vi "GUI_DG645_2.0.0.vi"() -> ()   [LabVIEW 2013]
uses:
  DelayControl_For Multiple Channels.ctl
  Device Drivers/DG645/subVIs/channels_TypDef.ctl
  DelayControl2.ctl
  Device Drivers/DG645/subVIs/polarity_TypDEf.ctl
  Shared/GUI_Template/GUI_master/tcp_new_data_event.ctl
  Shared/GUI_Template/GUI_master/tcp new data cluster.ctl
panel:
  out "tcp data event":T1
  in  "Refresh Button":bool
  in  "GUIdevice 1":string="P2-AndorCam"
  out "UDP error message":string caption="Device Errors"
  in  "Plot":bool
  in  "Tab Control":enum32{"All Channels", "Internal", "Advanced"}(tab)
  out "Plot Array":cluster{"Waveform Graph":dbl[]}[](array[cluster])
  in  "Amplitude.Ch GH::1":dbl=4.0 caption="Amplitude (V)" min=0.5 max=5.0
  in  "Amplitude.Ch T0::1":dbl=4.0 caption="Amplitude (V)" min=0.5 max=5.0
  in  "Polarity.Ch GH::1":T2=enum."Positive" caption="Polarity"
  in  "Polarity.Ch T0::1":T2=enum."Positive" caption="Polarity"
  in  "Delay.Ch T1":T3={"Channel"="T1", "Linked"=enum."T0", "Delay"=0.03} {"Delay" format="%+.12f"}
  in  "Delay.Ch T0":T3={"Channel"="T0", "Linked"=enum."T0", "Delay"=0.0} {"Delay" format="%+.12f"}
  in  "Delay.Ch H":T3={"Channel"="H", "Linked"=enum."G", "Delay"=0.03} {"Delay" format="%+.12f"}
  in  "Delay.Ch G":T3={"Channel"="G", "Linked"=enum."T0", "Delay"=0.0} {"Delay" format="%+.12f"}
  in  "Polarity.Ch EF::1":T2=enum."Positive" caption="Polarity"
  in  "Amplitude.Ch EF::1":dbl=4.0 caption="Amplitude (V)" min=0.5 max=5.0
  in  "Delay.Ch F":T3={"Channel"="F", "Linked"=enum."E", "Delay"=0.03} {"Delay" format="%+.12f"}
  in  "Delay.Ch E":T3={"Channel"="E", "Linked"=enum."T0", "Delay"=0.0} {"Delay" format="%+.12f"}
  in  "Polarity.Ch CD::1":T2=enum."Positive" caption="Polarity"
  in  "Amplitude.Ch CD::1":dbl=4.0 caption="Amplitude (V)" min=0.5 max=5.0
  in  "Delay.Ch D":T3={"Channel"="D", "Linked"=enum."C", "Delay"=0.03} {"Delay" format="%+.12f"}
  in  "Delay.Ch C":T3={"Channel"="C", "Linked"=enum."T0", "Delay"=0.0} {"Delay" format="%+.12f"}
  in  "Delay.Ch B":T3={"Channel"="B", "Linked"=enum."A", "Delay"=0.03} {"Delay" format="%+.12f"}
  in  "Delay.Ch A":T3={"Channel"="A", "Linked"=enum."T0", "Delay"=0.0} {"Delay" format="%+.12f"}
  in  "Amplitude.Ch AB:::1":dbl=3.0 caption="Amplitude (V)"
  in  "Polarity.Ch AB::1":T2=enum."Positive" caption="Polarity"
  in  "local saving path::1":path caption="Local Saving Path"
  in  "load file::1":bool caption="Load file"
  in  "save::1":bool caption="save"
  in  "trigger::1":bool caption="Trigger"
  in  "load local::1":T6(ring) caption="load local"
  in  "save local::1":T6(ring) caption="save local"
  in  "trigger.rate::1":dbl=10.0 caption="Rate (Hz)" min=0.001 max=1000.0
  in  "trigger.source::1":T7(ring)=enum."External rising edges" caption="Source"
  in  "Inhibit::1":T8(ring)=enum."Triggers" caption="Inhibit"
  in  "stop":bool
  # "AB"
  # "CD"
  # "EF"
  # "GH"
  # "T0"
  # "="
  # "="
  # "="
  # "="
  # "="
  # "="
  # "="
  # "="
  # "="
  # "="
  # "TRIGGER"
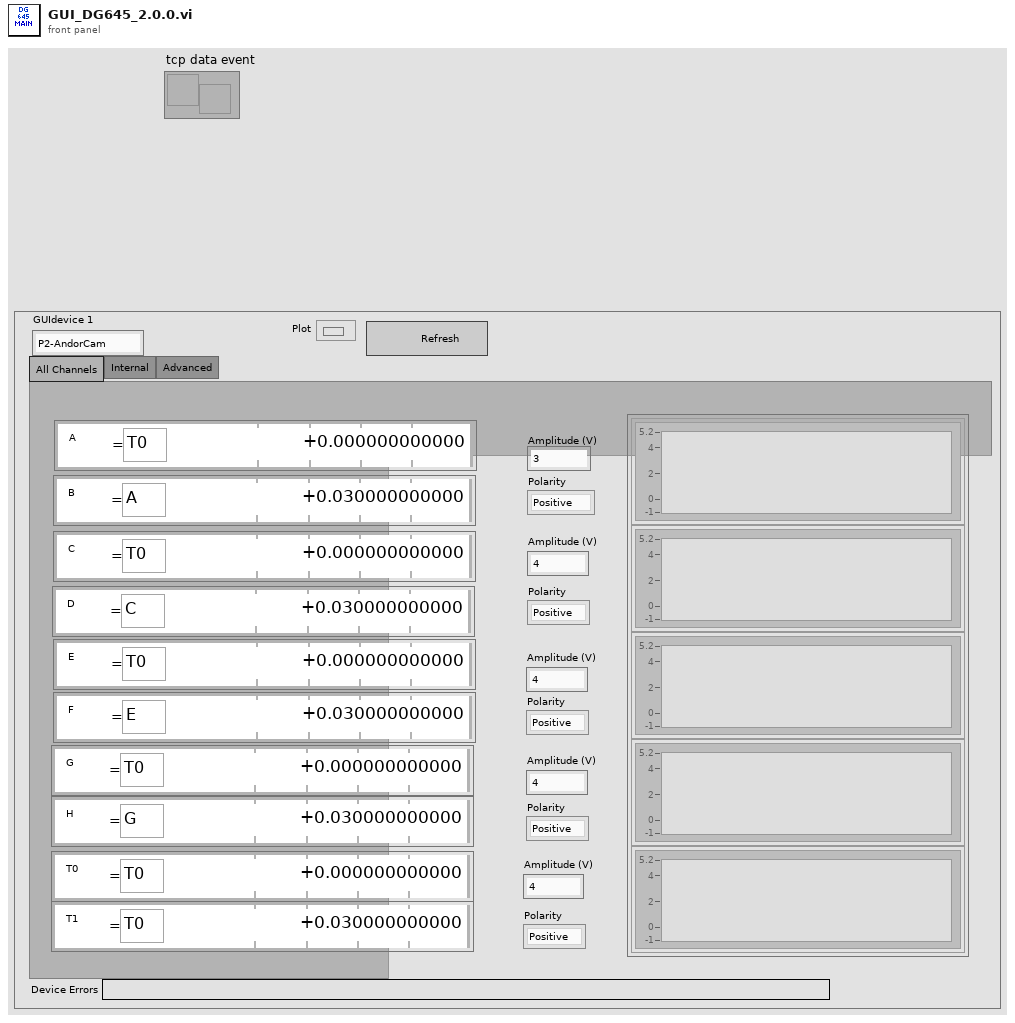
[diagram p1: front panel]
types:
  T1 = typedef "tcp_new_data_event.ctl" = refnum<user-event>
  T2 = typedef "polarity_TypDEf.ctl" = enum16{"Negative", "Positive"}
  T3 = typedef "DelayControl_For Multiple Channels.ctl" = cluster{"Channel":string, "Linked":T4, "Delay":T5}
  T4 = typedef "channels_TypDef.ctl" = enum16{"T0", "T1", "A", "B", "C", "D", "E", "F", "G", "H"}
  T5 = typedef "DelayControl2.ctl" = dbl
  T6 = enum16{"off", "1", "2", "3", "4", "5", "6", "7", "8", "9"}
  T7 = enum16{"Internal", "External rising edges", "External falling edges", "Single shot external rising edges", "Single shot external falling edges", "Single shot", "Line"}
  T8 = enum16{"off", "Triggers", "AB", "AB and CD", "AB, CD and EF", "AB, CD, EF and GH"}
  T9 = enum32{"invalid app kind", "Development System", "Run Time System", "Student Edition", "Embedded LabVIEW", "Evaluation", "Custom"}
  T10 = typedef "tcp new data cluster.ctl" = cluster{"EventEnum":enum16{"new data", "connection status update"}, "Device name":string}
  T11 = enum32{"Invalid", "Standard", "Closed", "Hidden", "Minimized", "Maximized"}
  T12 = cluster{"Core":cluster{"Current VI Reference":refnum<vi>, "Close Panel on Exit?":bool}, "Your Boolean data":bool, "Your string data":string, "SuperGUI":cluster{"STOP queue":refnum<queue>, "SuperGUI ref":refnum<vi>}}
  T13 = cluster{"STOP queue":refnum<queue>, "SuperGUI ref":refnum<vi>}
  T14 = cluster{"Current VI Reference":refnum<vi>, "Close Panel on Exit?":bool}
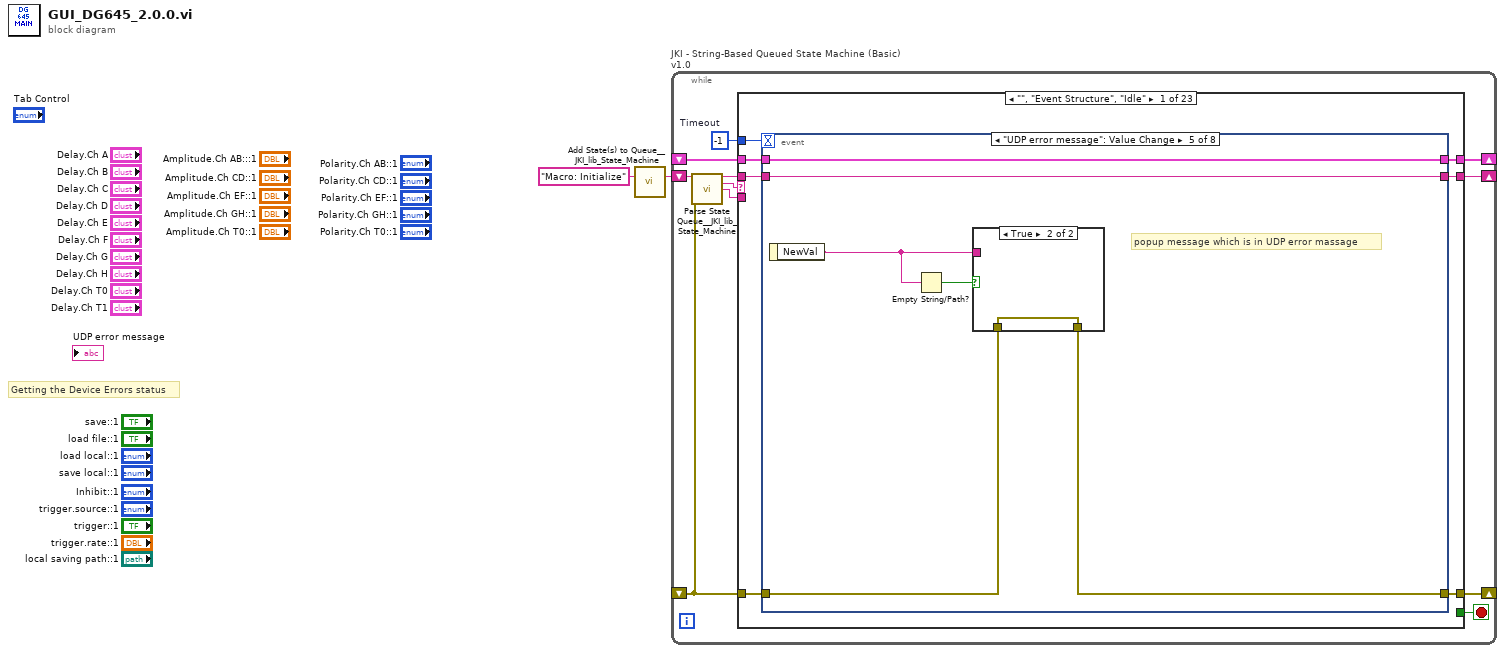
[diagram p0: block diagram]
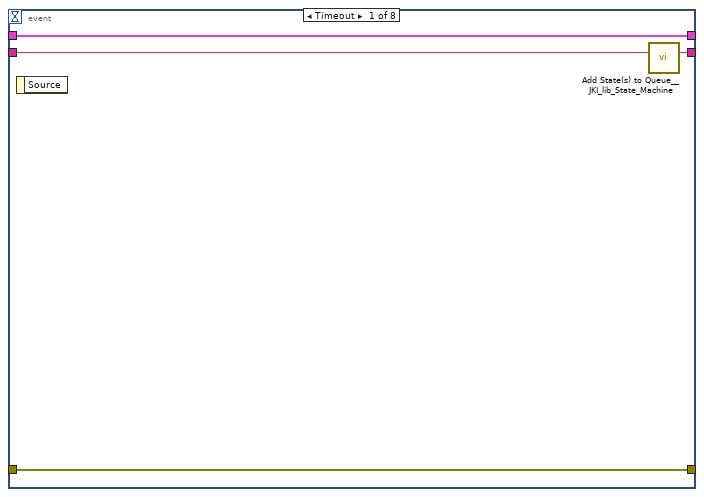
[diagram p2: hidden frame]
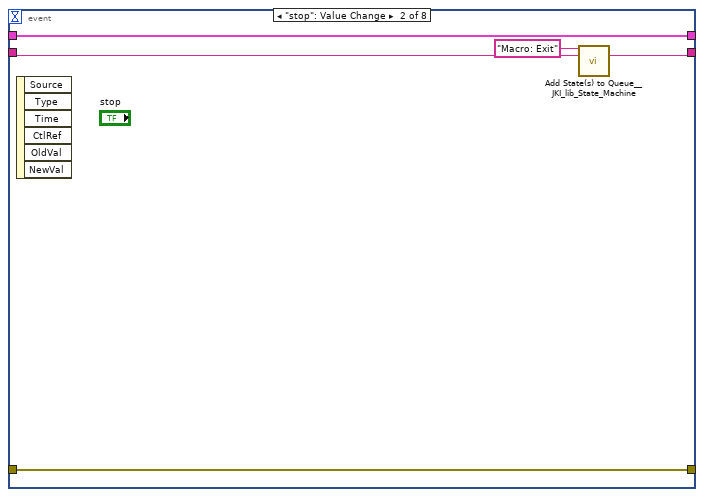
[diagram p3: hidden frame]
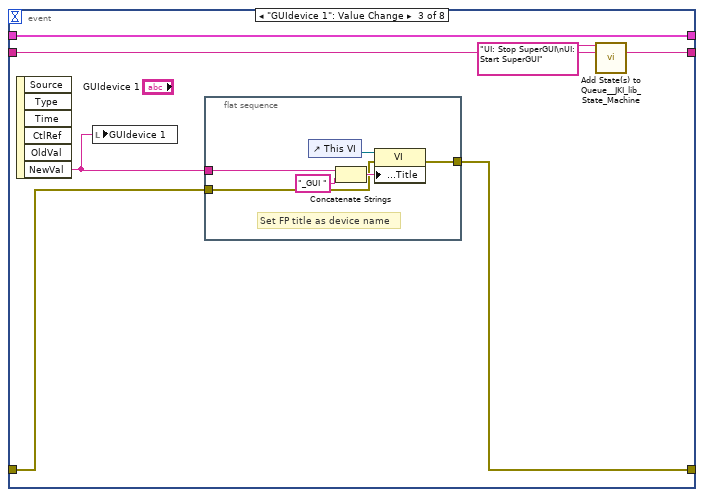
[diagram p4: hidden frame]
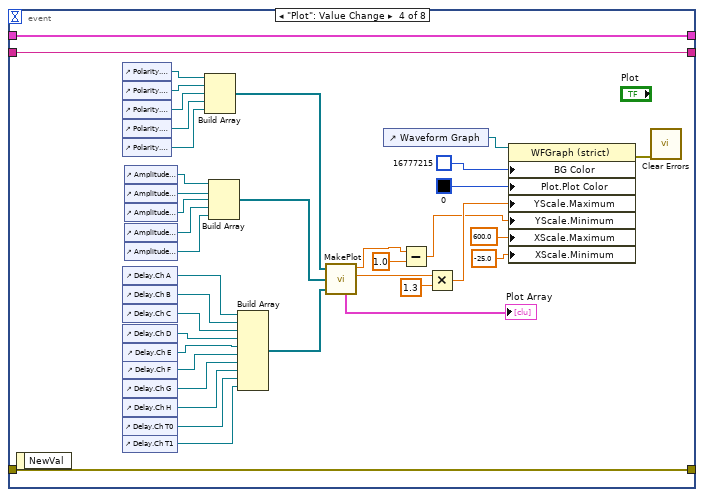
[diagram p5: hidden frame]
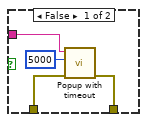
[diagram p6: hidden frame]
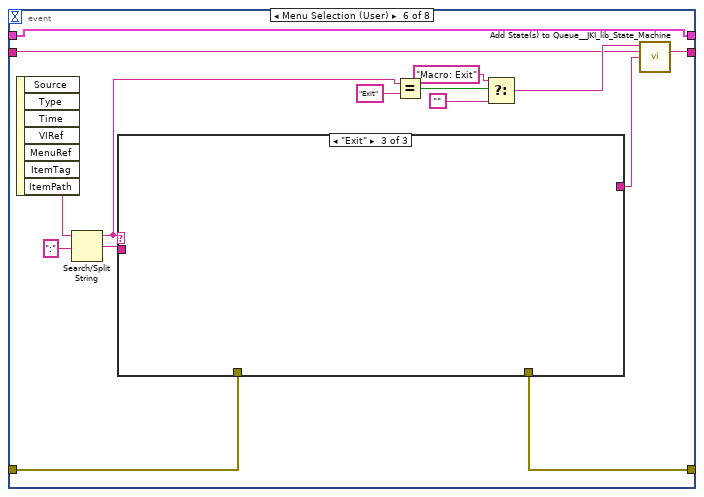
[diagram p7: hidden frame]
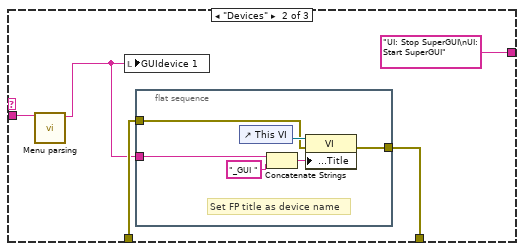
[diagram p9: hidden frame]
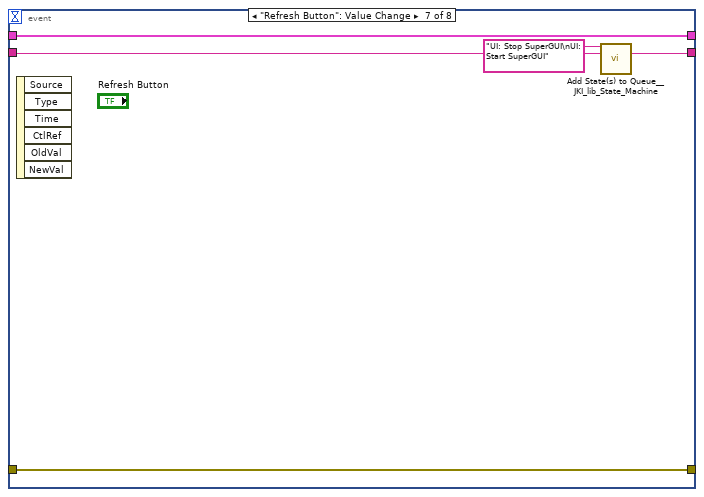
[diagram p10: hidden frame]
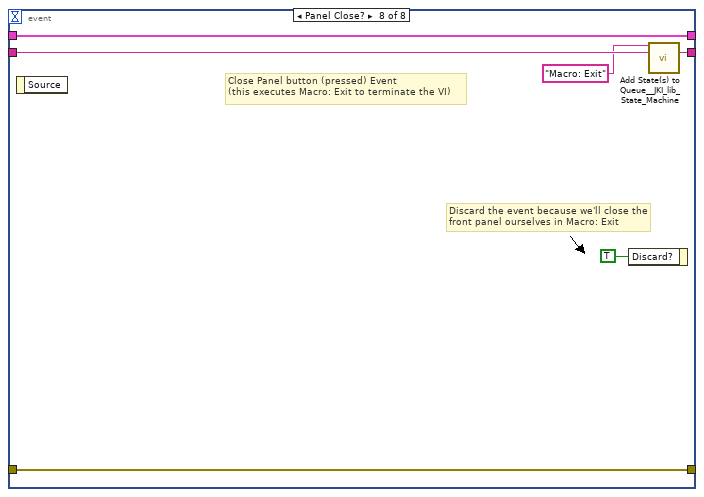
[diagram p11: hidden frame]
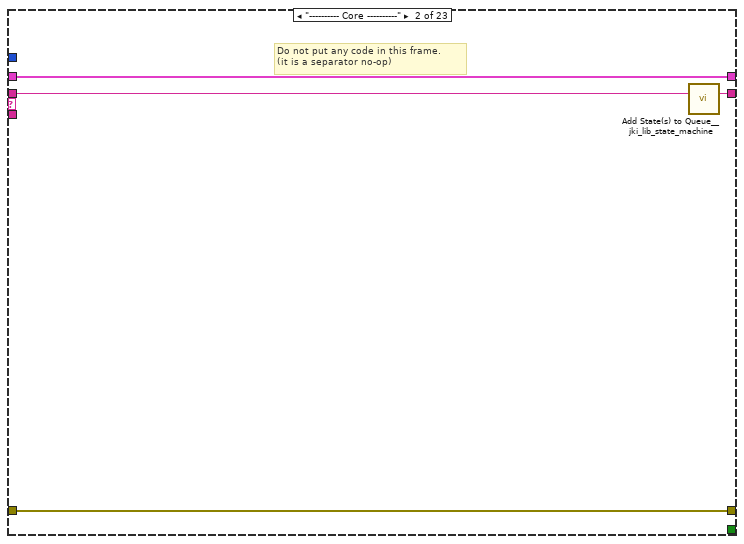
[diagram p12: hidden frame]
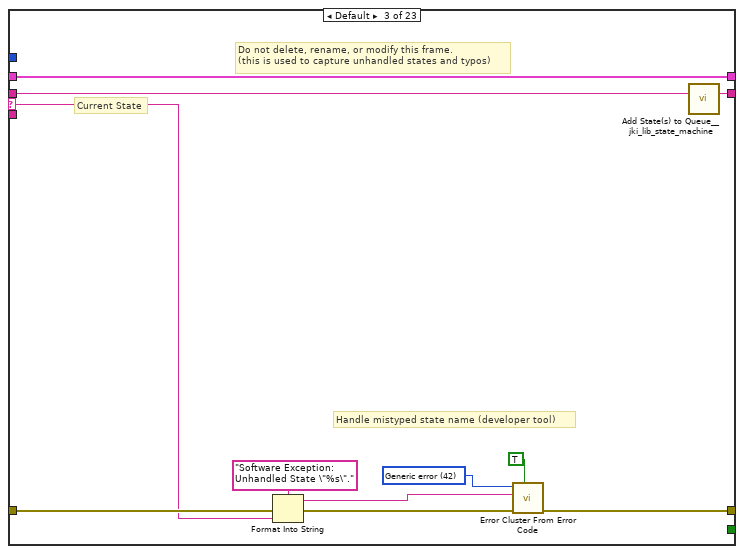
[diagram p13: hidden frame]
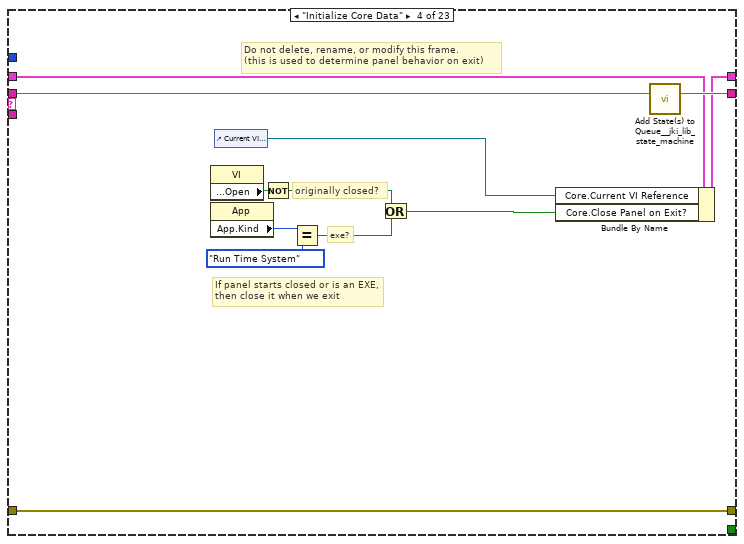
[diagram p14: hidden frame]
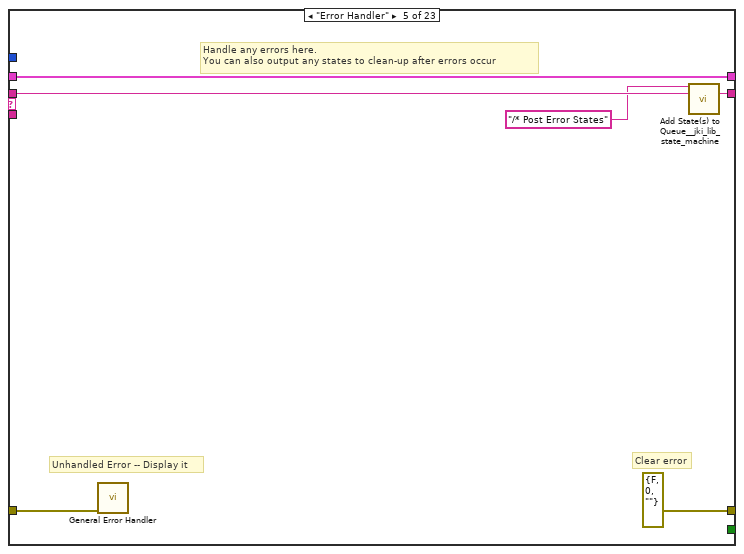
[diagram p15: hidden frame]
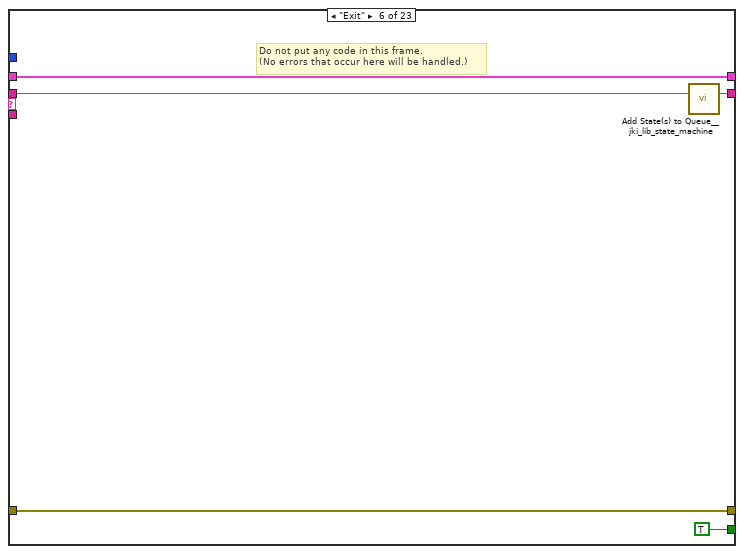
[diagram p16: hidden frame]
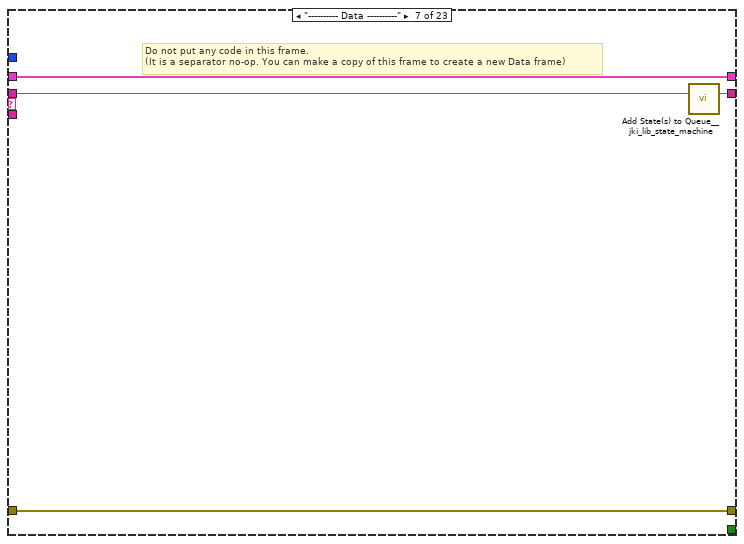
[diagram p17: hidden frame]
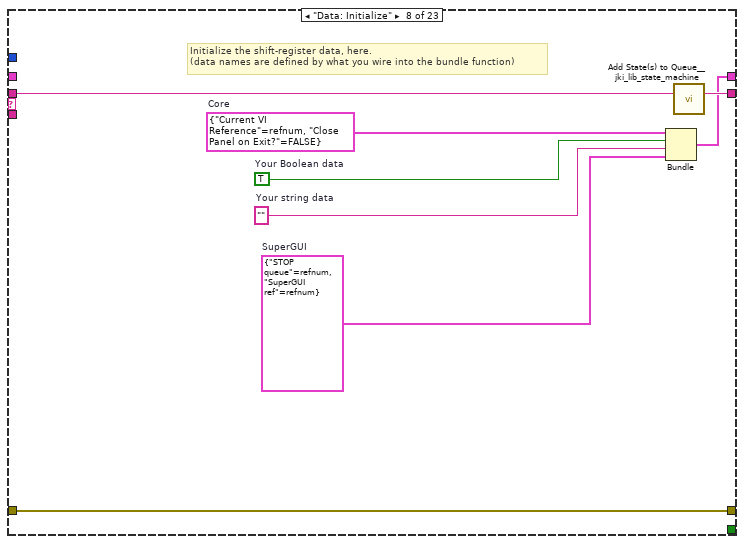
[diagram p18: hidden frame]
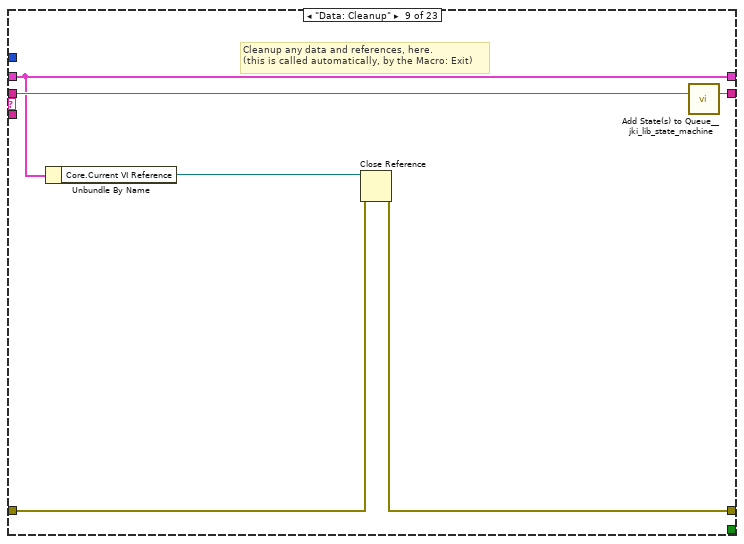
[diagram p19: hidden frame]
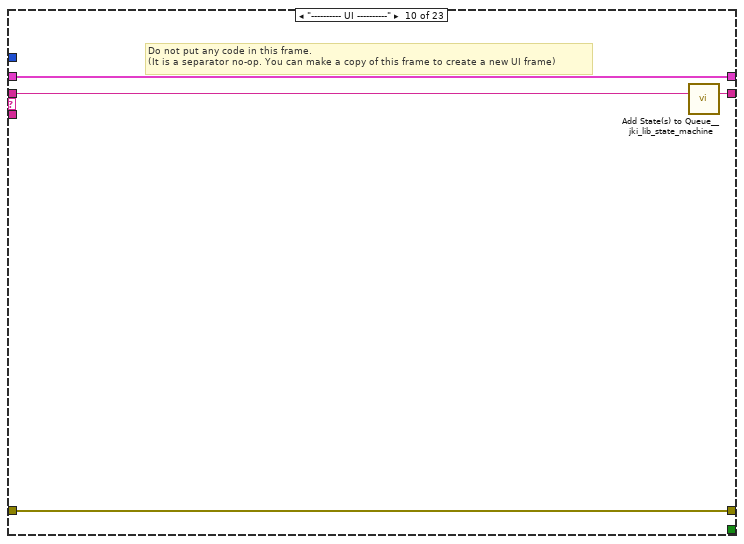
[diagram p20: hidden frame]
diagram:
  # "Getting the Device Errors status"
  n1 = call <vilib>:"Add State(s) to Queue__JKI_lib_State_Machine.vi"("State(s) in (\"\")"="Macro: Initialize") -> ("States Out"=w2:string)  [unwired: 14 in]
  n2 = while "JKI - String-Based Queued State Machine (Basic) v1.0" {
    shift-right: [w6] -> _
    shift-left: _ -> [w5]
    shift-right: [w9] -> _
    shift-left: _ -> [w3]
    shift-right: [w8] -> _
    shift-left: w2 -> [w10]
    stop <- w7 stop-if-true
    w4 = -1  # Timeout
    n3 = call <vilib>:"Parse State Queue__JKI_lib_State_Machine.vi"("State Queue"=w10, "Error In (no error)"=w3) -> ("Remaining States"=w12:string, "Current State"=w13:string, "Arguments"=w11:string)  [unwired: 11 in]
    n4 = case shown="\"\", \"Event Structure\", \"Idle\"" w13 {
      selector: w13 -> [_ _ w136 _ _ _ _ _ _ _ _ _ _ _ _ _ _ _ _ _ _ _ _]
      tunnel: w12 -> [w20 w135 w140 w158 w164 w169 w173 w181 w187 w191 w196 w204 w236 w270 w278 w284 w295 w321 w326 w336 w340 w344 w348]
      tunnel: w11 -> [_ _ _ _ _ _ _ _ _ _ _ _ _ _ _ w279 w289 _ _ _ _ _ _]
      tunnel: w5 -> [w18 w132 w138 w149 w161 w167 w170 _ w182 w188 w194 w202 w234 w261 w273 w282 w291 w318 w323 w333 w337 w341 w345]
      tunnel: [w17 w133 w142 w155 errorcluster {"status"=FALSE, "code"=0, "source"=""} ("error out") w166 w171 w178 w183 w189 w192 w200 w231 w254 w271 w280 w292 w319 w324 w334 w338 w342 w346] -> w9
      tunnel: w3 -> [w16 w133 w141 w155 w160 w166 w171 w178 w184 w189 w193 w201 w232 w255 w272 w281 w293 w319 w324 w334 w338 w342 w346]
      tunnel: [w19 w134 w139 w157 w163 w168 w172 w180 w186 w190 w195 w203 w235 w269 w277 w283 w294 w320 w325 w335 w339 w343 w347] -> w8
      tunnel: [_ _ _ _ _ TRUE _ _ _ _ _ _ _ _ _ _ _ _ _ _ _ _ _] -> w7
      tunnel: [w15 w132 w138 w156 w161 w167 w170 w179 w182 w188 w194 w202 w234 w260 w273 w282 w291 w318 w323 w333 w337 w341 w345] -> w6
      tunnel: w4 -> [w14 _ _ _ _ _ _ _ _ _ _ _ _ _ _ _ _ _ _ _ _ _ _]
      frame "", "Event Structure", "Idle" {
        n5 = event shown="[4] \"UDP error message\": Value Change" {
          selector: _ -> [_ _ _ _ _ _ _ _]
          dyn-events: _ -> [_ _ _ _ _ _ _ _]
          timeout: w14 -> [_ _ _ _ _ _ _ _]
          tunnel: w20 -> [w24 w27 w33 w80 w86 w101 w123 w131]
          tunnel: [w23 w26 w32 w80 w86 w100 w122 w130] -> w19
          tunnel: w18 -> [w21 w29 w36 w81 w87 w107 w125 w128]
          tunnel: [w22 w28 w34 w79 w82 w94 w124 w129] -> w17
          tunnel: w16 -> [w22 w28 w35 w79 w83 w95 w124 w129]
          tunnel: [w21 w29 w36 w81 w87 w107 w125 w128] -> w15
          event Timeout {
            n6 = event-data() -> ()  [unwired: 1 in, 1 out]
            n7 = call <vilib>:"Add State(s) to Queue__JKI_lib_State_Machine.vi"("State(s) in (\"\")"=w24) -> ("States Out"=w23:string)  [unwired: 14 in]
          }
          event "stop": Value Change {
            n8 = event-data() -> ()  [unwired: 1 in, 6 out]
            n9 = call <vilib>:"Add State(s) to Queue__JKI_lib_State_Machine.vi"("State(s) in Front (\"\")"="Macro: Exit", "State(s) in (\"\")"=w27) -> ("States Out"=w26:string)  [unwired: 13 in]
          }
          event "GUIdevice 1": Value Change {
            n10 = event-data() -> ("NewVal"=w30:string)  [unwired: 1 in, 5 out]
            n11 = local write "GUIdevice 1"(w30) -> ()
            n12 = flat-sequence {
              tunnel: [w39] -> w34
              tunnel: w35 -> [w38]
              tunnel: w30 -> [w37]
              frame #0 {
                # "Set FP title as device name"
                n13 = control-ref of="This VI"() -> (w42:refnum<vi>)
                n14 = Concatenate Strings(w37, "_GUI ") -> (w41:string)
                n15 = property class="VI"(reference=w42, error in=w38, "Front Panel.Title"=w41) -> (error out=w39:errorcluster)  [unwired: 1 out]
              }
            }
            n16 = call <vilib>:"Add State(s) to Queue__JKI_lib_State_Machine.vi"("State(s) in Front (\"\")"="UI: Stop SuperGUI\nUI: Start SuperGUI", "State(s) in (\"\")"=w33) -> ("States Out"=w32:string)  [unwired: 13 in]
          }
          event "Plot": Value Change {
            n17 = event-data() -> ()  [unwired: 1 in, 1 out]
            n18 = control-ref of="Polarity.Ch AB"() -> (w65:refnum<vi>)
            n19 = control-ref of="Polarity.Ch CD"() -> (w64:refnum<vi>)
            n20 = control-ref of="Polarity.Ch EF"() -> (w63:refnum<vi>)
            n21 = control-ref of="Polarity.Ch GH"() -> (w62:refnum<vi>)
            n22 = control-ref of="Polarity.Ch T0"() -> (w61:refnum<vi>)
            n23 = control-ref of="Delay.Ch A"() -> (w53:refnum<vi>)
            n24 = control-ref of="Delay.Ch B"() -> (w52:refnum<vi>)
            n25 = control-ref of="Delay.Ch C"() -> (w51:refnum<vi>)
            n26 = control-ref of="Delay.Ch D"() -> (w50:refnum<vi>)
            n27 = control-ref of="Delay.Ch E"() -> (w49:refnum<vi>)
            n28 = control-ref of="Delay.Ch F"() -> (w48:refnum<vi>)
            n29 = control-ref of="Delay.Ch G"() -> (w47:refnum<vi>)
            n30 = control-ref of="Delay.Ch H"() -> (w46:refnum<vi>)
            n31 = control-ref of="Delay.Ch T0"() -> (w45:refnum<vi>)
            n32 = control-ref of="Delay.Ch T1"() -> (w44:refnum<vi>)
            n33 = control-ref of="Amplitude.Ch AB:::1"() -> (w59:refnum<vi>)
            n34 = control-ref of="Amplitude.Ch CD::1"() -> (w58:refnum<vi>)
            n35 = control-ref of="Amplitude.Ch EF::1"() -> (w57:refnum<vi>)
            n36 = control-ref of="Amplitude.Ch GH::1"() -> (w56:refnum<vi>)
            n37 = control-ref of="Amplitude.Ch T0::1"() -> (w55:refnum<vi>)
            n38 = Build Array(w65, w64, w63, w62, w61) -> (w60:refnum<vi>[])
            n39 = Build Array(w59, w58, w57, w56, w55) -> (w54:refnum<vi>[])
            n40 = Build Array(w53, w52, w51, w50, w49, w48, w47, w46, w45, w44) -> (w43:refnum<vi>[])
            n41 = call "MakePlot.vi"("Polarity array"=w60, "Amplitude array"=w54, "Channel array"=w43) -> ("min value"=w69:dbl, "Numeric 3"=w74:dbl, "Array"=→"Plot Array":cluster{"Pulse Pattern":dbl[]}[])  [unwired: 2 out]
            n42 = control-ref of="Waveform Graph"() -> (w67:refnum<vi>)
            n43 = Subtract(x=w69, y=1.0) -> (x-y=w68:dbl)
            n44 = Multiply(x=w74, y=1.3) -> (x*y=w76:dbl)
            n45 = property class="WFGraph (strict)"(reference=w67, "BG Color"=u32 16777215 ("Color"), "Plot.Plot Color"=u32 0 ("Color"), "YScale.Maximum"=w76, "YScale.Minimum"=w68, "XScale.Maximum"=600.0 ("X Scale.Range:Maximum"), "XScale.Minimum"=-25.0 ("X Scale.Range:Minimum")) -> (error out=w70:errorcluster)  [unwired: 1 in, 1 out]
            n46 = call <vilib>:"Clear Errors.vi"("error in (no error)"=w70) -> ()  [unwired: 6 in, 1 out]
          }
          event "UDP error message": Value Change {
            # "popup message which is in UDP error massage"
            n47 = event-data() -> ("NewVal"=w84:string)  [unwired: 1 in]
            n48 = Empty String/Path?(string/path=w84) -> (empty?=w85:bool)
            n49 = case shown="True" w85 {
              tunnel: w84 -> [w91 _]
              tunnel: w83 -> [w90 w92]
              tunnel: [w89 w92] -> w82
              frame False {
                n50 = call "Popup with timeout.vi"("error"=w90, "timeout"=u32 5000, "message"=w91) -> ("error out"=w89:errorcluster)  [unwired: 8 in]
              }
              frame True {
              }
            }
          }
          event Menu Selection (User) {
            n51 = event-data() -> ("ItemPath"=w97:string)  [unwired: 1 in, 6 out]
            n52 = Search/Split String(string=w97, search string/char (-)=":") -> (substring before match=w93:string, match + rest of string=w96:string)  [unwired: 1 in, 1 out]
            n53 = case shown="\"Exit\"" w93 {
              tunnel: w96 -> [_ w113 _]
              tunnel: w95 -> [w108 w112 w120]
              tunnel: [w108 w111 w120] -> w94
              tunnel: [_ "UI: Stop SuperGUI\nUI: Start SuperGUI" _] -> w99
              frame "", Default {
              }
              frame "Devices" {
                n54 = call "Menu parsing.vi"("ItemPath 3"=w113) -> ("ItemPath 2"=w109:string)  [unwired: 9 in, 1 out]
                n55 = local write "GUIdevice 1"(w109) -> ()
                n56 = flat-sequence {
                  tunnel: [w116] -> w111
                  tunnel: w112 -> [w115]
                  tunnel: w109 -> [w114]
                  frame #0 {
                    # "Set FP title as device name"
                    n57 = control-ref of="This VI"() -> (w119:refnum<vi>)
                    n58 = Concatenate Strings(w114, "_GUI ") -> (w118:string)
                    n59 = property class="VI"(reference=w119, error in=w115, "Front Panel.Title"=w118) -> (error out=w116:errorcluster)  [unwired: 1 out]
                  }
                }
              }
              frame "Exit" {
              }
            }
            n60 = Equal?(x=w93, y="Exit") -> (x = y?=w105:bool)
            n61 = Select(t="Macro: Exit", s=w105, f="") -> (s? t:f=w102:string)
            n62 = call <vilib>:"Add State(s) to Queue__JKI_lib_State_Machine.vi"("State(s) in Front (\"\")"=w102, "State(s) in (\"\")"=w101, "State(s) at Back (\"\")"=w99) -> ("States Out"=w100:string)  [unwired: 12 in]
          }
          event "Refresh Button": Value Change {
            n63 = event-data() -> ()  [unwired: 1 in, 6 out]
            n64 = call <vilib>:"Add State(s) to Queue__JKI_lib_State_Machine.vi"("State(s) in Front (\"\")"="UI: Stop SuperGUI\nUI: Start SuperGUI", "State(s) in (\"\")"=w123) -> ("States Out"=w122:string)  [unwired: 13 in]
          }
          event Panel Close? {
            # "Discard the event because we'll close the front panel ourselves in Macro: Exit"
            # "Close Panel button (pressed) Event\n(this executes Macro: Exit to terminate the VI)"
            n65 = event-data() -> ()  [unwired: 1 in, 1 out]
            n66 = event-data("Discard?"=TRUE) -> ()  [unwired: 1 in, 1 out]
            n67 = call <vilib>:"Add State(s) to Queue__JKI_lib_State_Machine.vi"("State(s) in Front (\"\")"="Macro: Exit", "State(s) in (\"\")"=w131) -> ("States Out"=w130:string)  [unwired: 13 in]
          }
        }
      }
      frame "---------- Core ----------" {
        # "Do not put any code in this frame.\n(it is a separator no-op)"
        n68 = call <vilib>:"Add State(s) to Queue__jki_lib_state_machine.vi"("State(s) in (\"\")"=w135) -> ("States Out"=w134:string)  [unwired: 14 in]
      }
      frame Default {
        w145 = 42 items=["No error", "Argument error", "Memory is full", "Out of zone", "End of file", "File already open", "Generic file I/O error", "File not found", "File permission error", "Disk is full", "Duplicate path", "Too many files open", "System feature not enabled", "Resource file not found", "Cannot add resource", "Resource not found", "Image not found", "Image memory error", "Pen does not exist", "Config type invalid", "Config token not found", "Config parse error", "Config memory error", "Bad external code format", "Bad external code offset", "External code not present", "Null window", "Destroy window error", "Null menu", "Print aborted", "Bad print record", "Print driver error", "Windows error during printing", "Memory error during printing", "Print dialog error", "Generic print error", "Invalid device refnum", "Device not found", "Device parameter error", "Device unit error", "Cannot open device", "Device call aborted", "Generic error", "Cancelled by user", "Object ID too low", "Object ID too high", "Object not in heap", "Unknown heap", "Unknown object (invalid DefProc)", "Unknown object (DefProc not in table)", "Message out of range", "Invalid (null) method", "Unknown message", "Manager call not supported", "Bad address", "Network operation in progress", "Network operation timed out", "Connection is busy", "Network attribute not supported", "Network error", "Address in use", "System out of memory", "Connection aborted", "Connection refused", "Not connected", "Already connected", "Connection closed", "Initialization error (interapplication manager)", "Bad occurrence", "Wait on unbound occurrence handler", "Occurrence queue overflow", "Datalog type conflict", "Unused", "Unrecognized type (interapplication manager)", "Memory corrupt", "Failed to make temporary DLL", "Old CIN version", "Drag socket not found", "Failed to load drop-object", "Failed to register OLE object", "Failed to release OLE object", "Format specifier type mismatch", "Unknown format specifier", "Too few format specifiers", "Too many format specifiers", "Scan failed", "Newer CIN version", "Error converting to variant", "Runtime menu error", "Password tampered", "Variant attribute not found", "Incompatible variant data type", "Event data is not available", "Event Store is not present", "Occurrence is not found", "Event Queue is not created", "Event info is not available", "Refnum passed is NULL", "Error retrieving Class GUID", "Error retrieving CoClass GUID", "Error retrieving TypeLib GUID.", "Bad built application magic bytes.", "Specific driver is different from the specific driver associated with the Logical Name.", "There is no session opened to the class driver.", "Max Error", "MAX - Error with config objects", "MAX - Error loading configuration", "MAX - Group not supported"]
        # "Current State"
        # "Do not delete, rename, or modify this frame.\n(this is used to capture unhandled states and typos)"
        # "Handle mistyped state name (developer tool)"
        n69 = Format Into String(format string="Software Exception: Unhandled State \"%s\"." ("message"), error in=w141, w136) -> (resulting string=w144:string, error out=w143:errorcluster)  [unwired: 1 in]
        n70 = call <vilib>:"Error Cluster From Error Code.vi"("show call chain? (False)"=TRUE, "error in (no error)"=w143, "error message (\"\")"=w144, "error code (0)"=w145) -> ("error out"=w142:errorcluster)  [unwired: 5 in]
        n71 = call <vilib>:"Add State(s) to Queue__jki_lib_state_machine.vi"("State(s) in (\"\")"=w140) -> ("States Out"=w139:string)  [unwired: 14 in]
      }
      frame "Initialize Core Data" {
        # "Do not delete, rename, or modify this frame.\n(this is used to determine panel behavior on exit)"
        # "originally closed?"
        # "exe?"
        # "If panel starts closed or is an EXE, then close it when we exit"
        n72 = property class="VI"() -> ("Front Panel.Open"=w154:bool)  [unwired: 2 in, 2 out]
        n73 = property class="App"() -> ("App.Kind"=w153:T9)  [unwired: 2 in, 2 out]
        n74 = control-ref of="Current VI Reference"() -> (w147:refnum<vi>)
        n75 = Not(x=w154) -> (.not. x?=w151:bool)
        n76 = Equal?(x=w153, y=T9."Run Time System" ("Application:Kind")) -> (x = y?=w150:bool)
        n77 = Or(x=w151, y=w150) -> (x .or. y?=w148:bool)
        n78 = Bundle By Name(cluster=w149, "Core.Current VI Reference"=w147, "Core.Close Panel on Exit?"=w148) -> (w156:T12)
        n79 = call <vilib>:"Add State(s) to Queue__jki_lib_state_machine.vi"("State(s) in (\"\")"=w158) -> ("States Out"=w157:string)  [unwired: 14 in]
      }
      frame "Error Handler" {
        # "Unhandled Error -- Display it"
        # "Handle any errors here.\nYou can also output any states to clean-up after errors occur"
        # "Clear error"
        n80 = call <vilib>:"General Error Handler.vi"("error in (no error)"=w160) -> ()  [unwired: 10 in, 5 out]
        n81 = call <vilib>:"Add State(s) to Queue__jki_lib_state_machine.vi"("State(s) in Front (\"\")"="/* Post Error States", "State(s) in (\"\")"=w164) -> ("States Out"=w163:string)  [unwired: 13 in]
      }
      frame "Exit" {
        # "Do not put any code in this frame.\n(No errors that occur here will be handled.)"
        n82 = call <vilib>:"Add State(s) to Queue__jki_lib_state_machine.vi"("State(s) in (\"\")"=w169) -> ("States Out"=w168:string)  [unwired: 14 in]
      }
      frame "---------- Data ----------" {
        # "Do not put any code in this frame.\n(It is a separator no-op. You can make a copy of this frame to create a new Data frame)"
        n83 = call <vilib>:"Add State(s) to Queue__jki_lib_state_machine.vi"("State(s) in (\"\")"=w173) -> ("States Out"=w172:string)  [unwired: 14 in]
      }
      frame "Data: Initialize" {
        w174 = T13 {"STOP queue"=refnum, "SuperGUI ref"=refnum}  # SuperGUI
        w175 = T14 {"Current VI Reference"=refnum, "Close Panel on Exit?"=FALSE}  # Core
        w177 = TRUE  # Your Boolean data
        w176 = ""  # Your string data
        # "Initialize the shift-register data, here.\n(data names are defined by what you wire into the bundle function)"
        n84 = Bundle("Core"=w175, "Your Boolean data"=w177, "Your string data"=w176, "SuperGUI"=w174) -> (w179:T12)  [unwired: 1 in]
        n85 = call <vilib>:"Add State(s) to Queue__jki_lib_state_machine.vi"("State(s) in (\"\")"=w181) -> ("States Out"=w180:string)  [unwired: 14 in]
      }
      frame "Data: Cleanup" {
        # "Cleanup any data and references, here.\n(this is called automatically, by the Macro: Exit)"
        n86 = Unbundle By Name(w182) -> ("Core.Current VI Reference"=w185:refnum<vi>)
        n87 = Close Reference(reference=w185, error in (no error)=w184) -> (error out=w183:errorcluster)
        n88 = call <vilib>:"Add State(s) to Queue__jki_lib_state_machine.vi"("State(s) in (\"\")"=w187) -> ("States Out"=w186:string)  [unwired: 14 in]
      }
      frame "---------- UI ----------" {
        # "Do not put any code in this frame.\n(It is a separator no-op. You can make a copy of this frame to create a new UI frame)"
        n89 = call <vilib>:"Add State(s) to Queue__jki_lib_state_machine.vi"("State(s) in (\"\")"=w191) -> ("States Out"=w190:string)  [unwired: 14 in]
      }
      frame "UI: Initialize" {
        # "Initialize the User Interface, here.\n(this is called automatically, by the Macro: Init)"
        n90 = call <userlib>:"Fit VI window to Largest Dec__ogtk.vi"("error in (no error)"=w193) -> ("error out"=w192:errorcluster)  [unwired: 5 in, 1 out]
        n91 = call <vilib>:"Add State(s) to Queue__jki_lib_state_machine.vi"("State(s) in (\"\")"=w196) -> ("States Out"=w195:string)  [unwired: 14 in]
      }
      frame "UI: Update Device List" {
        # "menu is not set visible in vi properties"
        n92 = call "getDevices.vi"("Device Class"="DG645") -> ("All Devices"=w198:string[])
        n93 = Empty Array?(array=w198) -> (empty?=w199:bool)
        n94 = case shown="False" w199 {
          tunnel: w201 -> [w207 w230]
          tunnel: [w206 w230] -> w200
          tunnel: w198 -> [w205 _]
          frame False {
            n95 = Current VI's Menubar() -> (w210:refnum<k9>)
            n96 = Get Menu Item Info(7:"Devices" ("item tag"), 8:w207, 11:w210) -> (0:w216:errorcluster, 3:w212:refnum<k9>)  [unwired: 5 out]
            n97 = Set Menu Item Info(7:"Devices" ("item tag"), 8:w216, 9:TRUE ("enabled"), 11:w212) -> (0:w215:errorcluster, 3:w214:refnum<k9>)  [unwired: 3 in]
            n98 = First Call?() -> (First Call?: T/F=w208:bool)
            n99 = case shown="True" w208 {
              tunnel: w214 -> [_ w222]
              tunnel: w205 -> [_ w221]
              tunnel: w215 -> [w217 w219]
              tunnel: [w217 w218] -> w206
              frame False {
              }
              frame True {
                n100 = for {
                  tunnel: [w229] -> w223
                  tunnel: w221 -> [w227] mode=indexing
                  tunnel: w222 -> [w226]
                  tunnel: [w225] -> w220
                  tunnel: w219 -> [w224]
                  n101 = Insert Menu Items(5:"Devices" ("menu tag"), 6:w224, 7:w227, 8:w227, 9:w226) -> (0:w225:errorcluster, 3:w229:refnum<k9>)  [unwired: 1 in, 1 out]
                }
                n102 = Enable Menu Tracking(2:w220, 4:w223) -> (0:w218:errorcluster)  [unwired: 1 in, 1 out]
              }
            }
          }
          frame True {
          }
        }
        n103 = call <vilib>:"Add State(s) to Queue__jki_lib_state_machine.vi"("State(s) in (\"\")"=w204) -> ("States Out"=w203:string)  [unwired: 14 in]
      }
      frame "UI: Get Device Name" {
        n104 = First Call?() -> (First Call?: T/F=w233:bool)
        n105 = case shown="True" w233 {
          tunnel: w232 -> [w237 w239]
          tunnel: [w237 w238] -> w231
          frame False {
          }
          frame True {
            n106 = disable-structure "Get Device name from control for vi mode\nand command line arg for exe" shown="RUN_TIME_ENGINE==True" {
              disable-tunnel: w239 -> [_ w241]
              disable-tunnel: [_ w240] -> w238
              frame condition #0 (active) {
              }
              frame condition #1 {
                n107 = control-ref of="This Application"() -> (w249:refnum<vi>)
                n108 = property class="App"(reference=w249) -> ("App.Args"=w248:string[])  [unwired: 1 in, 2 out]
                n109 = Index Array(array=w248, index #1=1 ("index")) -> (element #1=w242:string)  [unwired: 2 in, 2 out]
                n110 = Empty String/Path?(string/path=w242) -> (empty?=w246:bool)
                n111 = control-ref of="This VI"() -> (w245:refnum<vi>)
                n112 = case shown="False" w246 {
                  tunnel: w242 -> [w250 _]
                  frame False {
                    n113 = local write "GUIdevice 1"(w250) -> ()
                  }
                  frame True {
                  }
                }
                n114 = Concatenate Strings(w242, "_GUI ") -> (w244:string)
                n115 = property class="VI"(reference=w245, error in=w241, "Front Panel.Title"=w244) -> (error out=w240:errorcluster)  [unwired: 1 out]
              }
            }
          }
        }
        n116 = call <vilib>:"Add State(s) to Queue__jki_lib_state_machine.vi"("State(s) in (\"\")"=w236) -> ("States Out"=w235:string)  [unwired: 14 in]
      }
      frame "UI: Start SuperGUI" {
        # "create stop queue for supergui and its clones"
        # "x100 abort will be dependent on caller VI\nx80 abort will be independent of caller vi, this will abort vi when labview is closed."
        # "Start SuperGUI asynchronous way"
        n117 = vi-ref "GUI_Master_subvi_reentrant_queues.vi"() -> (w253:refnum<vi>)
        n118 = property class="VI"(reference=w253) -> ("Path"=w252:path)  [unwired: 1 in, 2 out]
        n119 = Create User Event(user event datatype=T10 {"EventEnum"=enum."new data", "Device name"="Device name"} ("New Event"), error in=w255) -> (user event=w256:refnum<user-event>, error out=w262:errorcluster)
        "tcp data event" <- w256
        n120 = control-ref of="This Application"() -> (w259:refnum<vi>)
        n121 = control-ref of="This VI"() -> (w258:refnum<vi>)
        n122 = Open VI Reference(type specifier VI Refnum (for type only)=refnum<vi> refnum, vi path=w252, options=256) -> (vi reference=w268:refnum<vi>, error out=w267:errorcluster)  [unwired: 3 in]
        n123 = register-events(w256) -> ()  [unwired: 2 in, 2 out]
        n124 = call "supergui create stop queue.vi"() -> ("STOP Queue out"=w264:refnum<queue>)  [unwired: 11 in]
        n125 = Current VI's Menubar() -> (w257:refnum<k9>)
        n126 = call-by-ref "Start Asynchronous Call"(reference=w268, error in=w267, "STOP Queue in"=w264, "This Application"=w259, 8:"error in (no error)"=w262, "tcp data event"=w256, "Caller menu reference"=w257, "Caller VI ref"=w258) -> (reference out=w251:refnum<vi>, error out=w254:errorcluster)  [unwired: 5 in, 1 out]
        n127 = Bundle By Name(cluster=w261, "SuperGUI.SuperGUI ref"=w251, "SuperGUI.STOP queue"=w264) -> (w260:T12)
        n128 = call <vilib>:"Add State(s) to Queue__jki_lib_state_machine.vi"("State(s) in (\"\")"=w270) -> ("States Out"=w269:string)  [unwired: 14 in]
      }
      frame "UI: Stop SuperGUI" {
        # "Stop Supergui Clone and wait until it exit properly"
        n129 = Unbundle By Name(w273) -> ("SuperGUI.SuperGUI ref"=w275:refnum<vi>, "SuperGUI.STOP queue"=w274:refnum<queue>)
        n130 = Release Queue(queue=w274, error in (no error)=w272) -> (error out=w276:errorcluster)  [unwired: 1 in, 2 out]
        n131 = call-by-ref "Wait On Asynchronous Call"(reference=w275, error in=w276) -> ("error out"=w271:errorcluster)  [unwired: 11 in, 2 out]
        n132 = call <vilib>:"Add State(s) to Queue__jki_lib_state_machine.vi"("State(s) in (\"\")"=w278) -> ("States Out"=w277:string)  [unwired: 14 in]
      }
      frame "UI: Cursor Set" {
        # "Argument"
        # "Set and Unset Cursor Busy.\n(Usage: \"UI: Cursor Set >> Busy|Idle\")"
        n133 = case shown="\"Idle\", Default" w279 {
          tunnel: w281 -> [w286 w288]
          tunnel: [w285 w287] -> w280
          frame "Idle", Default {
            n134 = call <vilib>:"Unset Busy.vi"("error in (no error)"=w286) -> ("error out"=w285:errorcluster)  [unwired: 10 in]
          }
          frame "Busy" {
            n135 = call <vilib>:"Set Busy.vi"("error in (no error)"=w288) -> ("error out"=w287:errorcluster)  [unwired: 9 in, 1 out]
          }
        }
        n136 = call <vilib>:"Add State(s) to Queue__jki_lib_state_machine.vi"("State(s) in (\"\")"=w284) -> ("States Out"=w283:string)  [unwired: 14 in]
      }
      frame "UI: Front Panel State" {
        # "Argument"
        # "Set Front Panel Open or Closed\n(Usage: \"UI: Front Panel State >> Open|Close\")"
        n137 = Unbundle By Name(w291) -> ("Core.Current VI Reference"=w290:refnum<vi>)
        n138 = case shown="\"Close\"" w289 {
          tunnel: w293 -> [w299 w312]
          tunnel: [w301 w313] -> w292
          tunnel: w290 -> [w300 w310]
          frame "Open", Default {
            n139 = property class="VI"(reference=w300, error in=w299) -> (reference out=w297:refnum<vi>, error out=w298:errorcluster, "Front Panel.Open"=w296:bool)
            n140 = case shown="False" w296 {
              tunnel: [w304 w307] -> w301
              tunnel: w298 -> [w303 w307]
              tunnel: w297 -> [w302 _]
              frame False {
                n141 = invoke class="VI" method="FP.Open"(reference=w302, error in=w303, "Activate"=TRUE, "State"=T11."Standard") -> (error out=w304:errorcluster)  [unwired: 1 in, 4 out]
              }
              frame True {
              }
            }
          }
          frame "Close" {
            n142 = property class="VI"(reference=w310, error in=w312) -> (reference out=w309:refnum<vi>, error out=w311:errorcluster, "Front Panel.Open"=w308:bool)
            n143 = case shown="True" w308 {
              tunnel: [w314 w317] -> w313
              tunnel: w311 -> [w314 w316]
              tunnel: w309 -> [_ w315]
              frame False {
              }
              frame True {
                n144 = invoke class="VI" method="FP.Close"(reference=w315, error in=w316) -> (error out=w317:errorcluster)  [unwired: 1 in, 2 out]
              }
            }
          }
        }
        n145 = call <vilib>:"Add State(s) to Queue__jki_lib_state_machine.vi"("State(s) in (\"\")"=w295) -> ("States Out"=w294:string)  [unwired: 14 in]
      }
      frame "---------- Macro ----------" {
        # "Do not put any code in this frame.\n(It is a separator no-op. You can make a copy of this frame to create a new Macro frame)"
        n146 = call <vilib>:"Add State(s) to Queue__jki_lib_state_machine.vi"("State(s) in (\"\")"=w321) -> ("States Out"=w320:string)  [unwired: 14 in]
      }
      frame "Macro: Initialize" {
        # "Initialization Macro\n(This is called once, when the VI starts)"
        n147 = call <vilib>:"Add State(s) to Queue__jki_lib_state_machine.vi"("State(s) in Front (\"\")"="Data: Initialize\nInitialize Core Data\nUI: Initialize\nUI: Update Device List\nUI: Get Device Name\nUI: Start SuperGUI\nUI: Front Panel State >> Open", "State(s) in (\"\")"=w326) -> ("States Out"=w325:string)  [unwired: 13 in]
      }
      frame "Macro: Exit" {
        # "Exit Macro\n(This is called once, when the VI exits)"
        n148 = Unbundle By Name(w333) -> ("Core.Close Panel on Exit?"=w332:bool)
        n149 = Select(t="UI: Front Panel State >> Close", s=w332, f="") -> (s? t:f=w329:string)
        n150 = call <vilib>:"Add State(s) to Queue__jki_lib_state_machine.vi"("State(s) in (\"\")"=w329, "State(s) at Back (\"\")"="Data: Cleanup\nExit") -> ("States Out"=w327:string)  [unwired: 13 in]
        n151 = call <vilib>:"Add State(s) to Queue__jki_lib_state_machine.vi"("State(s) in Front (\"\")"=w327, "State(s) in (\"\")"=w336) -> ("States Out"=w335:string)  [unwired: 13 in]
      }
      frame "---------- New Category ----------" {
        # "Template Separator\n(You can make a copy of, or modify, this frame)"
        n152 = call <vilib>:"Add State(s) to Queue__jki_lib_state_machine.vi"("State(s) in (\"\")"=w340) -> ("States Out"=w339:string)  [unwired: 14 in]
      }
      frame "New Category: 1" {
        # "Your code here.\n(You can make a copy of, or modify, this frame)"
        n153 = call <vilib>:"Add State(s) to Queue__jki_lib_state_machine.vi"("State(s) in (\"\")"=w344) -> ("States Out"=w343:string)  [unwired: 14 in]
      }
      frame "New Category: 2" {
        # "Your code here.\n(You can make a copy of, or modify, this frame)"
        n154 = call <vilib>:"Add State(s) to Queue__jki_lib_state_machine.vi"("State(s) in (\"\")"=w348) -> ("States Out"=w347:string)  [unwired: 14 in]
      }
    }
  }
